vi "Set Points.vi"(1 "Input":dbl, 2 "Set Points FGV Selector":T2, 3 "Action":T1) -> (0 "Output":dbl)   [LabVIEW 2013]
uses:
  Set Points FGV Selector.ctl
  Action.ctl
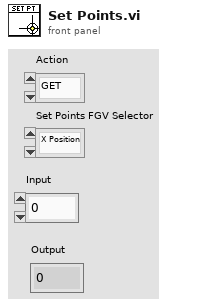
[diagram p1: front panel]
types:
  T1 = typedef "Action.ctl" = enum16{"GET", "PUT", "DELETE"}
  T2 = typedef "Set Points FGV Selector.ctl" = enum16{"X Position", "Y Position", "Z Position", "Z Scan"}
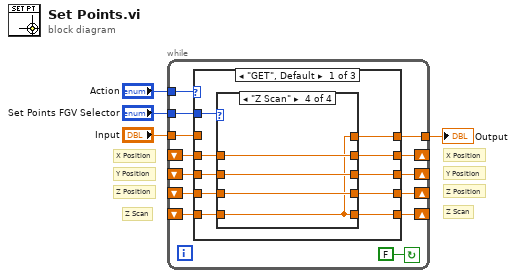
[diagram p0: block diagram]
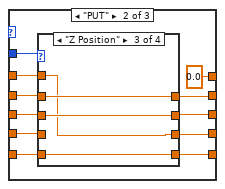
[diagram p5: hidden frame]
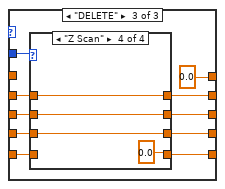
[diagram p9: hidden frame]
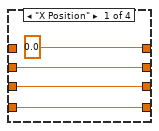
[diagram p10: hidden frame]
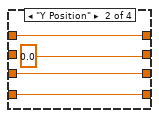
[diagram p11: hidden frame]
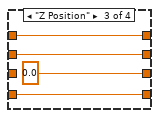
[diagram p12: hidden frame]
diagram:
  # "Z Scan"
  # "Z Scan"
  # "Z Position"
  # "Y Position"
  # "X Position"
  # "Z Position"
  # "Y Position"
  # "X Position"
  n1 = while {
    shift-right: [w14] -> _
    shift-left: _ -> [w13]
    shift-right: [w12] -> _
    shift-left: _ -> [w11]
    shift-right: [w10] -> _
    shift-left: _ -> [w9]
    tunnel: "Action" -> [w17]
    tunnel: "Set Points FGV Selector" -> [w16]
    tunnel: [w8] -> w2
    tunnel: "Input" -> [w7]
    shift-right: [w5] -> _
    shift-left: _ -> [w6]
    stop <- FALSE continue-if-true
    n2 = case shown="\"GET\", Default" w17 {
      tunnel: w16 -> [w27 w46 w73]
      tunnel: [w26 w51 w77] -> w14
      tunnel: w13 -> [w25 w54 w80]
      tunnel: [w24 w50 w76] -> w12
      tunnel: w11 -> [w23 w53 w79]
      tunnel: [w22 w49 w75] -> w10
      tunnel: w9 -> [w21 w52 w78]
      tunnel: [w20 0.0 0.0] -> w8
      tunnel: w7 -> [_ w47 _]
      tunnel: w6 -> [w19 w45 w71]
      tunnel: [w18 w44 w72] -> w5
      frame "GET", Default {
        n3 = case shown="\"Z Scan\"" w27 {
          tunnel: [w29 w35 w39 w43] -> w26
          tunnel: w25 -> [w29 w35 w39 w43]
          tunnel: [w31 w33 w38 w42] -> w24
          tunnel: w23 -> [w31 w33 w38 w42]
          tunnel: [w30 w34 w37 w41] -> w22
          tunnel: w21 -> [w30 w34 w37 w41]
          tunnel: [w29 w33 w37 w40] -> w20
          tunnel: w19 -> [w28 w32 w36 w40]
          tunnel: [w28 w32 w36 w40] -> w18
          frame "X Position" {
          }
          frame "Y Position" {
          }
          frame "Z Position" {
          }
          frame "Z Scan" {
          }
        }
      }
      frame "PUT" {
        n4 = case shown="\"Z Position\"" w46 {
          tunnel: [w56 w62 w66 w67] -> w51
          tunnel: w54 -> [_ w62 w66 w67]
          tunnel: [w58 w60 w65 w68] -> w50
          tunnel: w53 -> [w58 _ w65 w68]
          tunnel: [w57 w61 w64 w69] -> w49
          tunnel: w52 -> [w57 w61 _ w69]
          tunnel: w47 -> [w56 w60 w64 w70]
          tunnel: w45 -> [w55 w59 w63 _]
          tunnel: [w55 w59 w63 w70] -> w44
          frame "X Position" {
          }
          frame "Y Position" {
          }
          frame "Z Position" {
          }
          frame "Z Scan" {
          }
        }
      }
      frame "DELETE" {
        n5 = case shown="\"Z Scan\"" w73 {
          tunnel: [0.0 w88 w92 w96] -> w77
          tunnel: w80 -> [_ w88 w92 w96]
          tunnel: [w84 0.0 w91 w95] -> w76
          tunnel: w79 -> [w84 _ w91 w95]
          tunnel: [w83 w87 0.0 w94] -> w75
          tunnel: w78 -> [w83 w87 _ w94]
          tunnel: [w81 w85 w89 0.0 ("Input")] -> w72
          tunnel: w71 -> [w81 w85 w89 _]
          frame "X Position" {
          }
          frame "Y Position" {
          }
          frame "Z Position" {
          }
          frame "Z Scan" {
          }
        }
      }
    }
  }
  "Output" <- w2
